vi "OCUtoSim.vi"() -> ()   [LabVIEW 2011]
panel:
  in  "Wind Speed":dbl
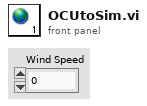
[diagram p1: front panel]
diagram:
